vi "SwerveMathTest_Luke.vi"() -> ()   [LabVIEW 2018]
panel:
  in  "Value at Forward Position":dbl=0.75 format="%#_13g"
  out "Theta Current":dbl format="%_4g"
  in  "Poteniometer":dbl(knob) scale=0.0..1.0
  out "Angular Distance (deg)":dbl format="%_4g"
  in  "Goal Angle":cluster{dbl, dbl}(knob)={0.0, 26.292506044716276} scale=180.0..-180.0
  # "forward is at 0.25 right now"
  # "goal is blue\ncurrent is orange"
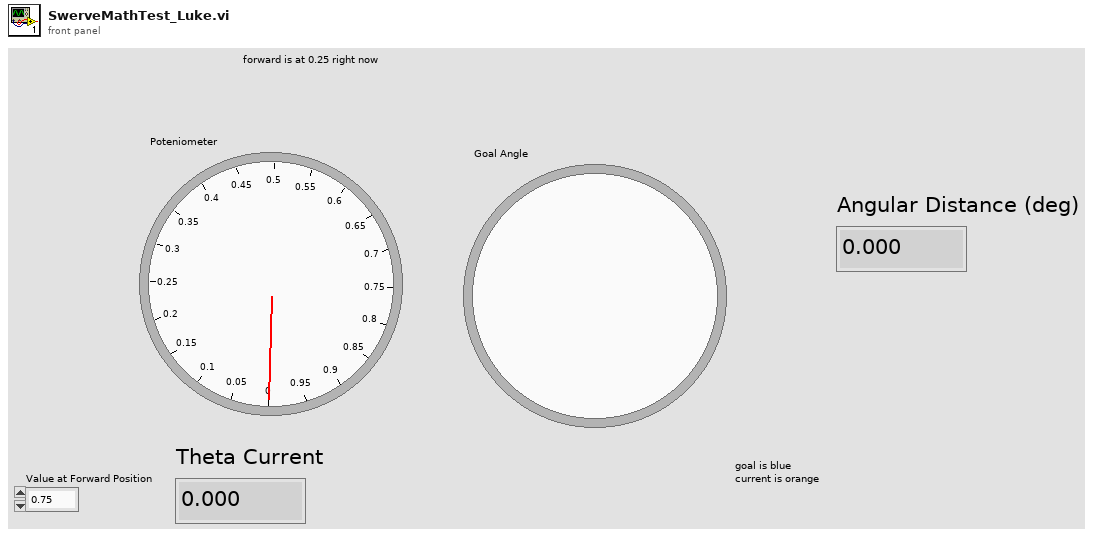
[diagram p1: front panel]
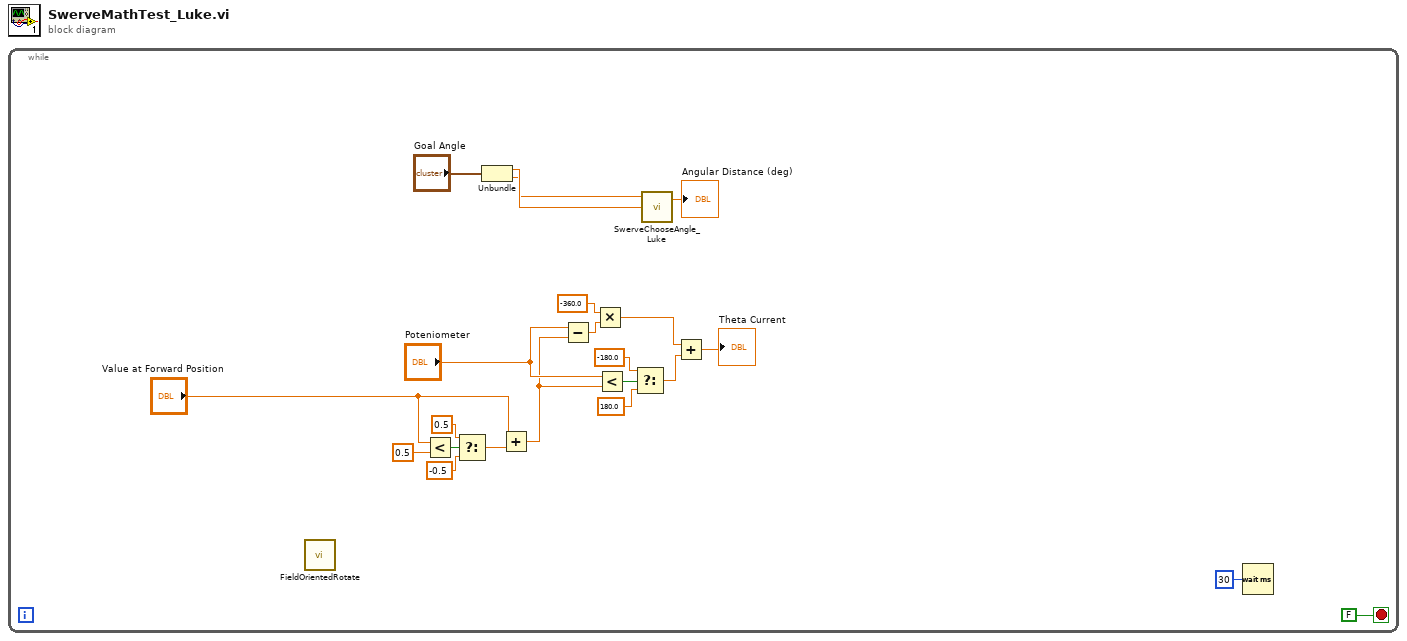
[diagram p0: block diagram]
diagram:
  n1 = while {
    stop <- FALSE stop-if-true
    n2 = call "FieldOrientedRotate.vi"() -> ()  [unwired: 4 in, 2 out]
    n3 = Less?(x="Value at Forward Position", y=0.5) -> (x < y?=w4:bool)
    n4 = Select(t=0.5 ("x"), s=w4, f=-0.5 ("x")) -> (s? t:f=w1:dbl)
    n5 = Unbundle("Goal Angle") -> (w18:dbl, w17:dbl)
    n6 = Add(x="Value at Forward Position", y=w1) -> (x+y=w7:dbl)
    n7 = Subtract(x="Poteniometer", y=w7) -> (x-y=w15:dbl)
    n8 = Multiply(x=-360.0, y=w15) -> (x*y=w14:dbl)
    n9 = Less?(x="Poteniometer", y=w7) -> (x < y?=w10:bool)
    n10 = Select(t=-180.0, s=w10, f=180.0) -> (s? t:f=w13:dbl)
    n11 = call "SwerveChooseAngle_Luke.vi"("Goal Angle (deg)"=w18, "Current Angle (deg)"=w17) -> ("Angular Distance (deg)"=→"Angular Distance (deg)":dbl)  [unwired: 1 in, 1 out]
    n12 = Add(x=w14, y=w13) -> (x+y=→"Theta Current":dbl)
    n13 = Wait (ms)(milliseconds to wait=u32 30) -> ()  [unwired: 1 out]
  }
